vi "convertMFCOutputBytes.vi"(8 "FullScale":dbl=24576.0, 9 "SCCM":dbl=500.0, 11 "Setpoint":dbl) -> (3 "Bytes":u8[](array[numeric]))   [LabVIEW 2011]
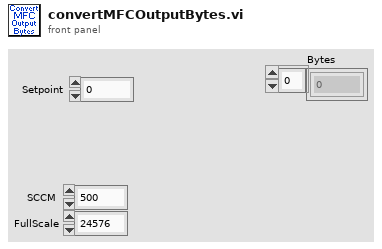
[diagram p1: front panel]
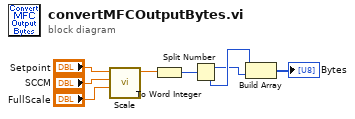
[diagram p0: block diagram]
diagram:
  n1 = call "Scale.vi"("Factor"="FullScale", "FullScale"="SCCM", "Input"="Setpoint") -> ("Output"=w5:dbl)  [unwired: 8 in]
  n2 = To Word Integer(number=w5) -> (16bit integer=w4:i16)
  n3 = Split Number(x=w4) -> (hi(x)=w2:u8, lo(x)=w3:u8)
  n4 = Build Array(w3, w2) -> (→"Bytes":u8[])
